vi "Turn.vi"(4 "lower limit":dbl, 6 "upper limit":dbl, 8 "error in":errorcluster, 11 "PID gains":T1) -> (0 "error out":errorcluster)   [LabVIEW 2016]
uses:
  <vilib>/addons/control/pid/pid.llb/PID (DBL).vi
  Robot Global Data.vi
  <vilib>/addons/control/pid/NI_PID_pid.lvlib
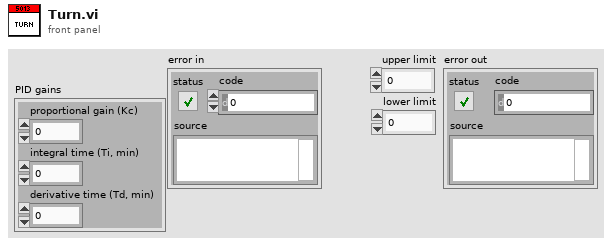
[diagram p1: front panel]
types:
  T1 = cluster{"proportional gain (Kc)":dbl, "integral time (Ti, min)":dbl, "derivative time (Td, min)":dbl}
  T2 = cluster{"Yaw":dbl, "Roll":dbl, "Pitch":dbl, "Heading":dbl, "Fused Heading":dbl}
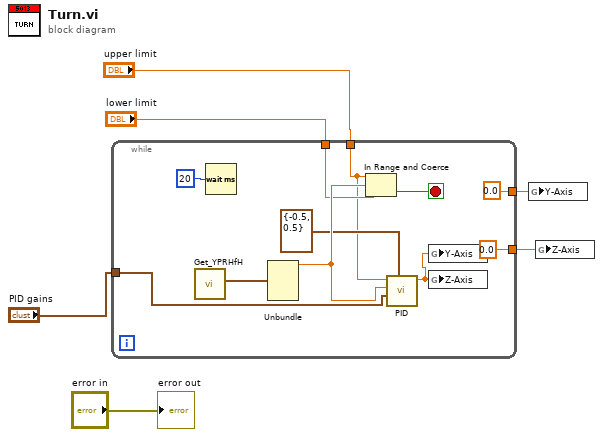
[diagram p0: block diagram]
diagram:
  n1 = while {
    tunnel: "PID gains" -> [w13]
    tunnel: "upper limit" -> [w9]
    tunnel: "lower limit" -> [w11]
    tunnel: [0.0 ("setpoint")] -> w2
    tunnel: [0.0 ("Y-Axis")] -> w1
    stop <- w16 stop-if-true
    n2 = call <vilib>:"Get_YPRHfH.vi"() -> ("YRPHfH"=w17:T2)  [unwired: 11 in]
    n3 = Wait (ms)(milliseconds to wait=u32 20) -> ()  [unwired: 1 out]
    n4 = Unbundle(w17) -> ("Yaw"=w14:dbl)  [unwired: 4 out]
    n5 = In Range and Coerce(upper limit=w9, x=w14, lower limit=w11) -> (In Range?=w16:bool)  [unwired: 1 out]
    n6 = call-poly <vilib>:"PID.vi"("output range"=cluster{"output high":dbl, "output low":dbl} {"output high"=-0.5, "output low"=0.5}, "PID gains"=w13, "process variable"=w14, "setpoint"=w9) -> ("output"=w7:dbl)  [unwired: 6 in, 1 out]
    n7 = global write "Robot Global Data.vi" "Y-Axis"(w7) -> ()
    n8 = global write "Robot Global Data.vi" "Z-Axis"(w7) -> ()
  }
  n9 = global write "Robot Global Data.vi" "Y-Axis"(w1) -> ()
  n10 = global write "Robot Global Data.vi" "Z-Axis"(w2) -> ()
  "error out" <- "error in"
